vi "hasPacketIdentifier.vi"(11 "PUBCOMP in":refnum<class "PUBCOMP.lvclass">) -> (2 "Has Packet Identifier":bool, 3 "PUBCOMP out":refnum<class "PUBCOMP.lvclass">)   [LabVIEW 2013, in "MQTT_Control_Packets.lvlib" / "PUBCOMP.lvclass"]
uses:
  PUBCOMP.lvclass
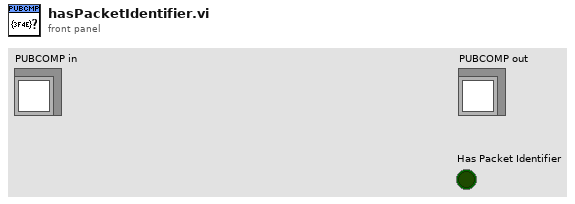
[diagram p1: front panel]
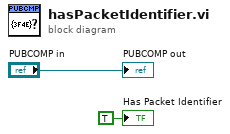
[diagram p0: block diagram]
diagram:
  "PUBCOMP out" <- "PUBCOMP in"
  "Has Packet Identifier" <- TRUE ("As Packet Identifier")
